vi "Capability Query.vi"(8 "error in (no error)":errorcluster, 11 "Refnum In":refnum<vi>) -> (0 "error out":errorcluster, 2 "Board Capability":map{i32, T1}(c390), 3 "Refnum Out":refnum<vi>)   [LabVIEW 2020]
doc: "Retrieve the capability of all the pins of the currently connected board. This mainly includes the list of modes supported by each pin along with the resolution for the mode (i.e. a Pin supporting Analog Mode might have a resolution of 14bits)"
uses:
  Controls/FirmataPinCapabilitiesAndAnalogMapping.ctl
  Controls/FirmataPinCapability.ctl
  FirmataClient.v1/controls/FirmataPinModes.ctl
  FirmataClient.v1/FirmataClient.lvlib
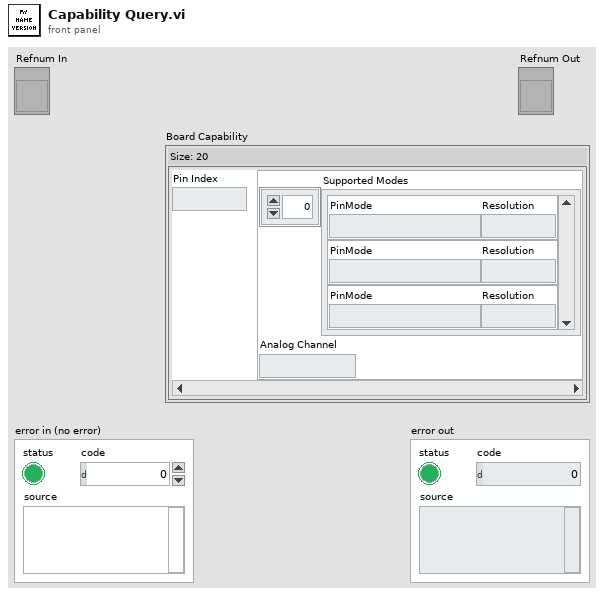
[diagram p1: front panel]
types:
  T1 = typedef "FirmataPinCapabilitiesAndAnalogMapping.ctl" = cluster{"Supported Modes":T2[], "Analog Channel":u8}
  T2 = typedef "FirmataPinCapability.ctl" = cluster{"PinMode":T3, "Resolution":u8}
  T3 = typedef "FirmataClient.lvlib/FirmataPinModes.ctl" = enum16{"DigitalInput", "DigitalOutput", "AnalogInput", "PWM", "Servo", "Shift", "I2C", "OneWire", "Stepper", "Encoder", "Serial", "InputPullup", "Extended.SPI", "Extended.Sonar", "Extended.Tone", "Extended.DHT"}
  T4 = typedef "FirmataProtocolConstants.ctl" = u16
  T5 = typedef "Parameters.ctl" = cluster{"Transport Parameters":T6, "Board Capabilities":map{i32, T1}}
  T6 = typedef "TransportParameters.ctl" = cluster{"Serial Communication":cluster{"Comport":refnum<visa-resource-name>, "No Response Timeout Ms":u32, "Response Complete Timeout Ms":u32, "Max Rx Length":u32, "Baud Rate":u32}, "Selected Transport":T7, "Initializer File Path":path, "Cleaner File Path":path, "Transporter File Path":path}
  T7 = typedef "SupportedTransports.ctl" = enum16{"Serial Communication Port"}
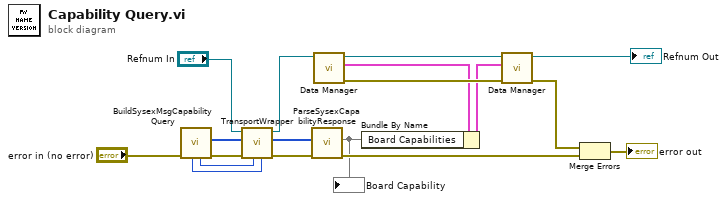
[diagram p0: block diagram]
diagram:
  n1 = call "BuildSysexMsgCapabilityQuery.vi"("error in"="error in (no error)") -> ("error out"=w18:errorcluster, "GetCapabilitiesMessage"=w13:u8[], "ReplyFirstByte"=w15:T4, "ReplyLength"=w14:i32)  [unwired: 7 in]
  n2 = call "TransportWrapper.vi"("ReplyLength"=w14, "ReplyFirstByte"=w15, "error in"=w18, "Message In"=w13, "Refnum In"="Refnum In") -> ("error out"=w12:errorcluster, "Message Out"=w11:u8[], "Refnum Out"=w10:refnum<vi>)  [unwired: 4 in]
  n3 = call "ParseSysexCapabilityResponse.vi"("error in"=w12, "Sysex Message"=w11) -> ("error out"=w5:errorcluster, "Map"=w2:map{i32, T1})  [unwired: 7 in, 1 out]
  "Board Capability" <- w2
  n4 = call "Data Manager.vi"("Refnum In"=w10) -> ("error out"=w7:errorcluster, "Data Out"=w3:T5, "Refnum Out"=w9:refnum<vi>)  [unwired: 8 in]
  n5 = Bundle By Name(cluster=w3, "Board Capabilities"=w2) -> (w1:T5)
  n6 = call "Data Manager.vi"("error in (no error)"=w7, "Data In"=w1, "Refnum In"=w9) -> ("error out"=w6:errorcluster, "Refnum Out"=→"Refnum Out":refnum<vi>)  [unwired: 6 in, 1 out]
  n7 = Merge Errors(w6, w5) -> (→"error out":errorcluster)
